vi "GetComputerHWInfo.vi"(11 "错误输入（无错误）":errorcluster, 12 "获取内容":enum16{"ALL", "HDD SN", "HDD Type", "MAC Adr"}(ring)) -> (8 "UID":string, 15 "error out":errorcluster)   [LabVIEW 2015]
uses:
  <vilib>/Utility/error.llb/whitespace.ctl
  <vilib>/regexp/Match Regular Expression.xnode
panel:
  out "BoardSN":string
  out "CPUID":string
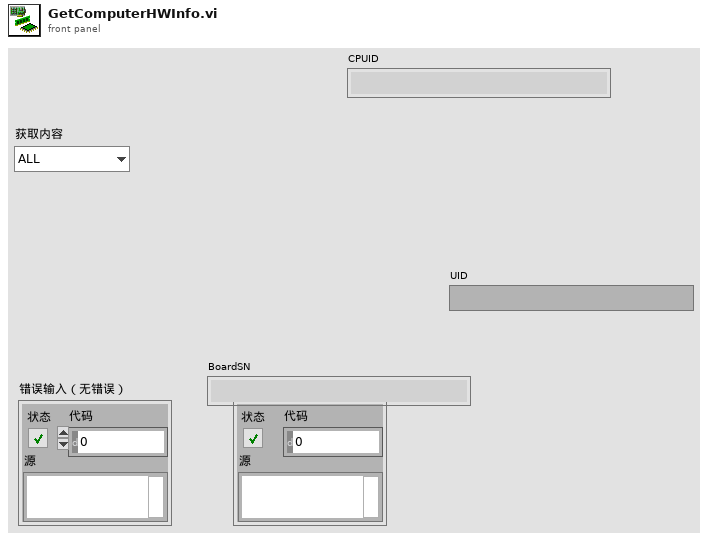
[diagram p1: front panel]
types:
  T1 = typedef "whitespace.ctl" = u16
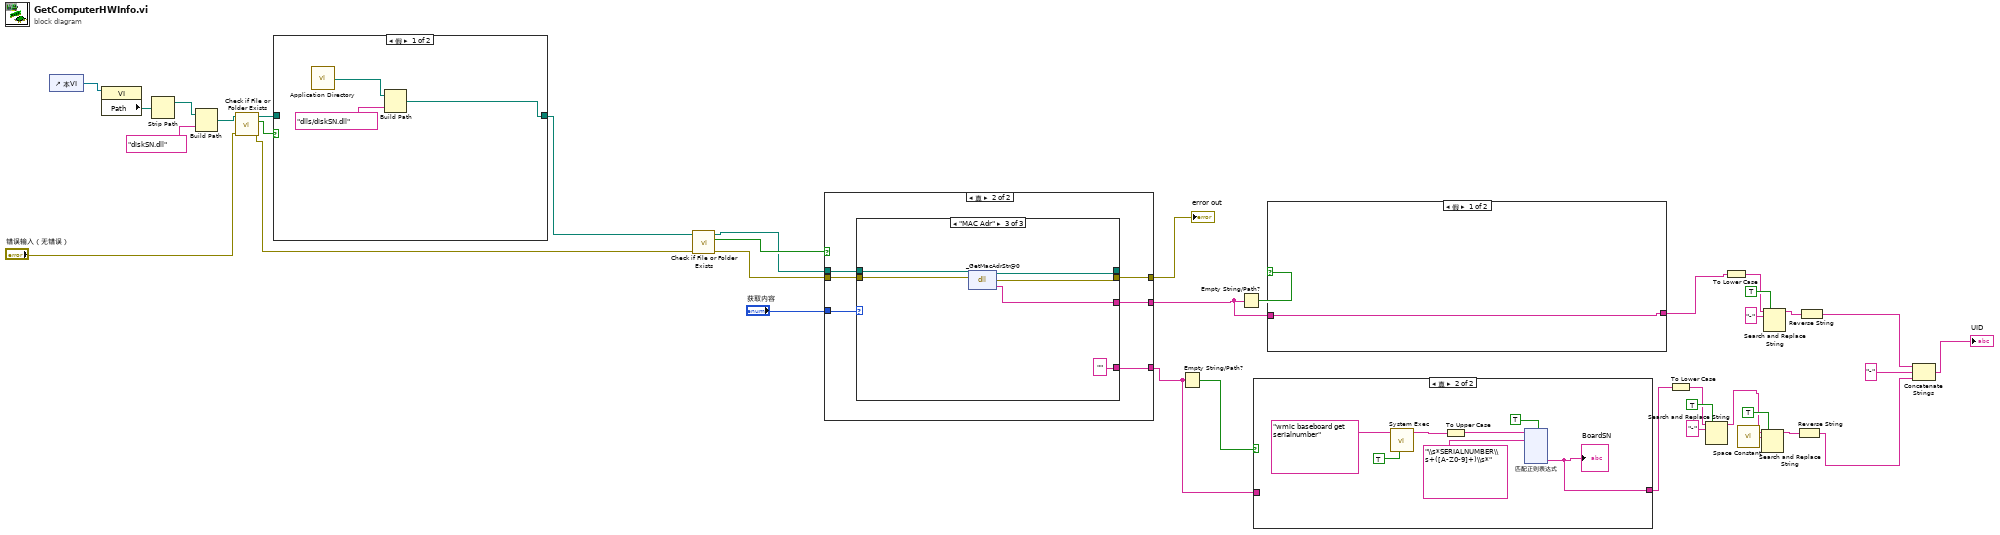
[diagram p0: block diagram]
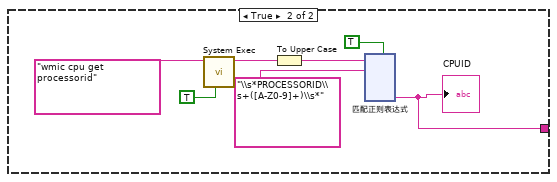
[diagram p3: hidden frame]
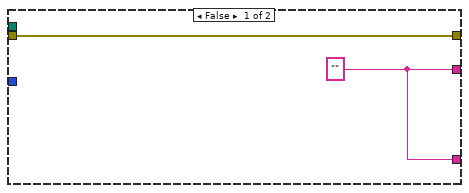
[diagram p5: hidden frame]
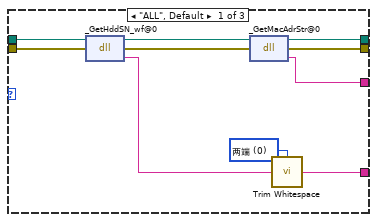
[diagram p6: hidden frame]
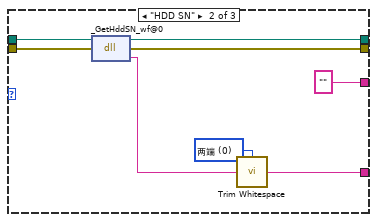
[diagram p7: hidden frame]
diagram:
  n1 = control-ref of="本VI"() -> (w34:refnum<vi>)
  n2 = property class="VI"(reference=w34) -> ("Path"=w33:path)  [unwired: 1 in, 2 out]
  n3 = Strip Path(path=w33) -> (stripped path=w32:path)  [unwired: 1 out]
  n4 = Build Path(base path=w32, name or relative path="diskSN.dll" ("名称或相对路径")) -> (appended path=w15:path)
  n5 = call <vilib>:"Check if File or Folder Exists.vi"("error in (no error)"="错误输入（无错误）", "path"=w15) -> ("error out"=w7:errorcluster, "file or folder exists?"=w14:bool, "dup path"=w13:path)  [unwired: 7 in]
  n6 = case shown="假" w14 {
    tunnel: w13 -> [_ w40]
    tunnel: [w37 w40] -> w11
    frame False {
      n7 = call <vilib>:"Application Directory.vi"() -> ("Application Directory"=w39:path)
      n8 = Build Path(base path=w39, name or relative path="dlls/diskSN.dll" ("名称或相对路径")) -> (appended path=w37:path)
    }
    frame True {
    }
  }
  n9 = call <vilib>:"Check if File or Folder Exists.vi"("error in (no error)"=w7, "path"=w11) -> ("error out"=w6:errorcluster, "file or folder exists?"=w10:bool, "dup path"=w9:path)  [unwired: 7 in]
  n10 = case shown="真" w10 {
    tunnel: "获取内容" -> [_ w48]
    tunnel: w6 -> [w42 w47]
    tunnel: [w41 w46] -> w4
    tunnel: [w41 w45] -> w2
    tunnel: [w42 w44] -> w35
    tunnel: w9 -> [_ w43]
    frame False {
      w41 = "" ("返回类型")
    }
    frame True {
      n11 = case shown="\"MAC Adr\"" w48 {
        tunnel: [w56 "" ("返回类型") w70] -> w46
        tunnel: [w53 w62 w71] -> w44
        tunnel: w47 -> [w55 w64 w72]
        tunnel: [w54 w63 "" ("trimmed string")] -> w45
        tunnel: w43 -> [w52 w60 w69]
        tunnel: [w51 w59 w68] -> _
        frame "ALL", Default {
          w58 = T1 0 items=["两端", "字符串首端", "字符串末端"] ("location (both)")
          n12 = dll-call lib="PTH2\\abs F\nWork Files开发软件资料[00] Labview[2] 收集de子VIdiskSN\ndiskSN.dll" fn="_GetHddSN_wf@0"(path in=w52, error in=w55) -> (path out=w50:path, error out=w49:errorcluster, "返回类型"=w57:string)  [unwired: 1 in]
          n13 = dll-call lib="PTH2\\abs F\nWork Files开发软件资料[00] Labview[2] 收集de子VIdiskSN\ndiskSN.dll" fn="_GetMacAdrStr@0"(path in=w50, error in=w49) -> (path out=w51:path, error out=w53:errorcluster, "返回类型"=w56:string)  [unwired: 1 in]
          n14 = call <vilib>:"Trim Whitespace.vi"("string"=w57, "location (both)"=w58) -> ("trimmed string"=w54:string)
        }
        frame "HDD SN" {
          w65 = T1 0 items=["两端", "字符串首端", "字符串末端"] ("location (both)")
          n15 = dll-call lib="PTH2\\abs F\nWork Files开发软件资料[00] Labview[2] 收集de子VIdiskSN\ndiskSN.dll" fn="_GetHddSN_wf@0"(path in=w60, error in=w64) -> (path out=w59:path, error out=w62:errorcluster, "返回类型"=w66:string)  [unwired: 1 in]
          n16 = call <vilib>:"Trim Whitespace.vi"("string"=w66, "location (both)"=w65) -> ("trimmed string"=w63:string)
        }
        frame "MAC Adr" {
          n17 = dll-call lib="PTH2\\abs F\nWork Files开发软件资料[00] Labview[2] 收集de子VIdiskSN\ndiskSN.dll" fn="_GetMacAdrStr@0"(path in=w69, error in=w72) -> (path out=w68:path, error out=w71:errorcluster, "返回类型"=w70:string)  [unwired: 1 in]
        }
      }
    }
  }
  "error out" <- w35
  n18 = Empty String/Path?(string/path=w2) -> (empty?=w3:bool)
  n19 = Empty String/Path?(string/path=w4) -> (empty?=w12:bool)
  n20 = case shown="真" w3 {
    tunnel: [w73 w74] -> w1
    tunnel: w2 -> [w73 _]
    frame False {
    }
    frame True {
      n21 = call <vilib>:"System Exec.vi"("run minimized? (F)"=TRUE, "command line"="wmic baseboard get serialnumber") -> ("standard output"=w77:string)  [unwired: 6 in, 3 out]
      n22 = To Upper Case(1:w77) -> (0:w80:string)
      n23 = xnode "匹配正则表达式"("输入字符串"=w80, "正则表达式"="\\s*SERIALNUMBER\\s+([A-Z0-9]+)\\s*", "多行？(F)"=TRUE) -> ("子匹配 1"=w74:string)  [unwired: 3 in, 5 out]
      "BoardSN" <- w74
    }
  }
  n24 = case shown="假" w12 {
    tunnel: [w197 w198] -> w5
    tunnel: w4 -> [w197 _]
    frame False {
    }
    frame True {
      n25 = call <vilib>:"System Exec.vi"("run minimized? (F)"=TRUE, "command line"="wmic cpu get processorid") -> ("standard output"=w201:string)  [unwired: 6 in, 3 out]
      n26 = To Upper Case(1:w201) -> (0:w202:string)
      n27 = xnode "匹配正则表达式"("输入字符串"=w202, "正则表达式"="\\s*PROCESSORID\\s+([A-Z0-9]+)\\s*", "多行？(F)"=TRUE) -> ("子匹配 1"=w198:string)  [unwired: 3 in, 5 out]
      "CPUID" <- w198
    }
  }
  n28 = To Lower Case(string=w1) -> (all lower case string=w24:string)
  n29 = Search and Replace String(replace all?=TRUE ("替换全部？(F)"), input string=w24, search string="-" ("搜索字符串")) -> (result string=w21:string)  [unwired: 5 in, 3 out]
  n30 = To Lower Case(string=w5) -> (all lower case string=w27:string)
  n31 = call <vilib>:"Space Constant.vi"() -> ("String"=w22:string)
  n32 = Search and Replace String(replace all?=TRUE ("替换全部？(F)"), input string=w21, search string=w22) -> (result string=w20:string)  [unwired: 5 in, 3 out]
  n33 = Search and Replace String(replace all?=TRUE ("替换全部？(F)"), input string=w27, search string="-" ("搜索字符串")) -> (result string=w28:string)  [unwired: 5 in, 3 out]
  n34 = Reverse String(1:w20) -> (0:w16:string)
  n35 = Reverse String(1:w28) -> (0:w17:string)
  n36 = Concatenate Strings(w17, "-" ("字符串"), w16) -> (→"UID":string)
